vi "Init Station V.vi"(8 "error in (no error)":errorcluster) -> (0 "error out":errorcluster, 3 "function return":i16)   [LabVIEW 2012, in "VantagePro.lvlib"]
doc: "DllAccess short int _stdcall InitStation_V(void);"
uses:
  VantagePro.lvlib
  VantagePro.dll
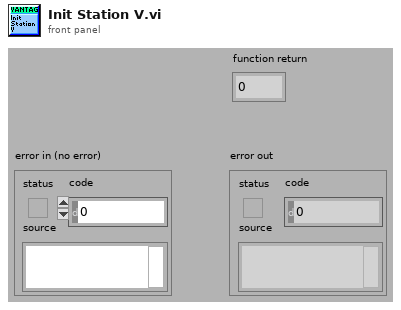
[diagram p1: front panel]
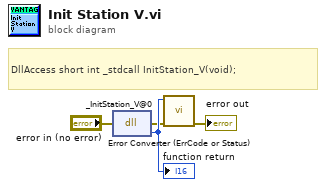
[diagram p0: block diagram]
diagram:
  # "DllAccess short int _stdcall InitStation_V(void);"
  n1 = dll-call lib="C:/Users/Dimitris/Desktop/BRITE/libs/VantagePro/VantagePro.*" fn="_InitStation_V@0"(error in="error in (no error)") -> (error out=w2:errorcluster, w4:i16)  [unwired: 2 in, 1 out]
  "function return" <- w4
  n2 = call "Error Converter (ErrCode or Status).vi"("error in (no error)"=w2, "error code"=w4) -> ("error out"=→"error out":errorcluster)  [unwired: 9 in]
